vi "AddMany.vi"(7 "Priority":refnum<class "Action.lvclass">[](array[class]), 11 "Stack in":refnum<class "Stack.lvclass">) -> (3 "Stack out":refnum<class "Stack.lvclass">)   [LabVIEW 2024, in "ActionStack.lvlib" / "Stack.lvclass"]
uses:
  Stack.lvclass
  Action/Action.lvclass
  Stack.lvclass/Stack.ctl
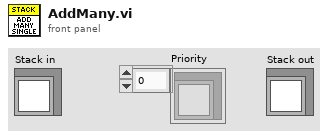
[diagram p1: front panel]
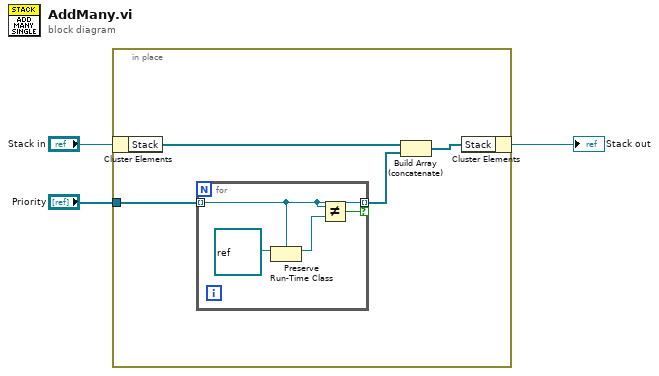
[diagram p0: block diagram]
diagram:
  n1 = in-place {
    in-place-border: "Priority" -> [w7]
    n2 = in-place-cluster #1("Stack in") -> ("Stack"=w6:refnum<class "Action.lvclass">[])
    n3 = for {
      tunnel: w7 -> [w9] mode=indexing
      tunnel: [w9] -> w5 mode=indexing if=w8
      n4 = Preserve Run-Time Class(object in=refnum<class> refnum, 2:w9) -> (object out=w10:refnum<class "Action.lvclass">)  [unwired: 1 in, 1 out]
      n5 = Not Equal?(x=w9, y=w10) -> (x != y?=w8:bool)
    }
    n6 = Build Array (concatenate)(w6, w5) -> (w4:refnum<class "Action.lvclass">[])
    n7 = in-place-cluster #1("Stack"=w4) -> (→"Stack out":refnum<class "Stack.lvclass">)
  }
